vi "Dark Sky Time Machine Request.vi"(0 "API Key":string, 1 "Units":T4="auto", 5 "Latitude":dbl=42.3601 min=-90.0 max=90.0, 7 "Longitude":dbl=-71.0589 min=-180.0 max=180.0, 9 "Time Machine Date/Time":timestamp=timestamp(3584408400 s since 1904-01-01), 11 "error in":errorcluster, 12 "Language":T5=enum."English") -> (4 "Time Machine Forecast Output":T3 {"Current Data"."currently"."time" format="%#_10g"}, 15 "error out":errorcluster)   [LabVIEW 2017, in "Dark Sky Weather Data for LabVIEW.lvlib"]
doc: "Makes a Time Machine request to the DarkSky API and interprets the result. A Time Machine request returns the observed (in the past) or forecasted (in the future) hour-by-hour weather and daily weather conditions for a particular date. Results include the overall data for the day, data by the hour of that day, and the current data for the specific minute, of the request, in that day.\n\nThis API call requires an API key (available free from DarkSky), latitude + longitude coordinates, and a date/time which can be in the past, present, or future. Use this alongside another API, for example from Google, to convert city names into coordinates if needed.\n\nMore info at https://darksky.net/dev/docs/time-machine\n\nNeed an API Key? Visit: https://darksky.net/dev/ and sign up for free!"
uses:
  Dark Sky Weather Data for LabVIEW.lvlib
  Controls/Language Enum.ctl
  Controls/Units Enum.ctl
  Controls/Lat_Lon_TZ.ctl
  Controls/Forecast Current Data.ctl
  <vilib>/httpClient/LabVIEWHTTPClient.lvlib
panel:
  out "API Call URL":string
  # "Inputs"
  # "Outputs - More Info at https://darksky.net/dev/docs/time-machine"
  # "Powered by Dark Sky"
  # "Need an API Key? Visit:\nhttps://darksky.net/dev/\nand sign up for free!"
  # "Instructions:\n-Enter an API Key\n-Enter Longitude, Latitude\n-Enter a Past UNIX Time\n-Run the VI"
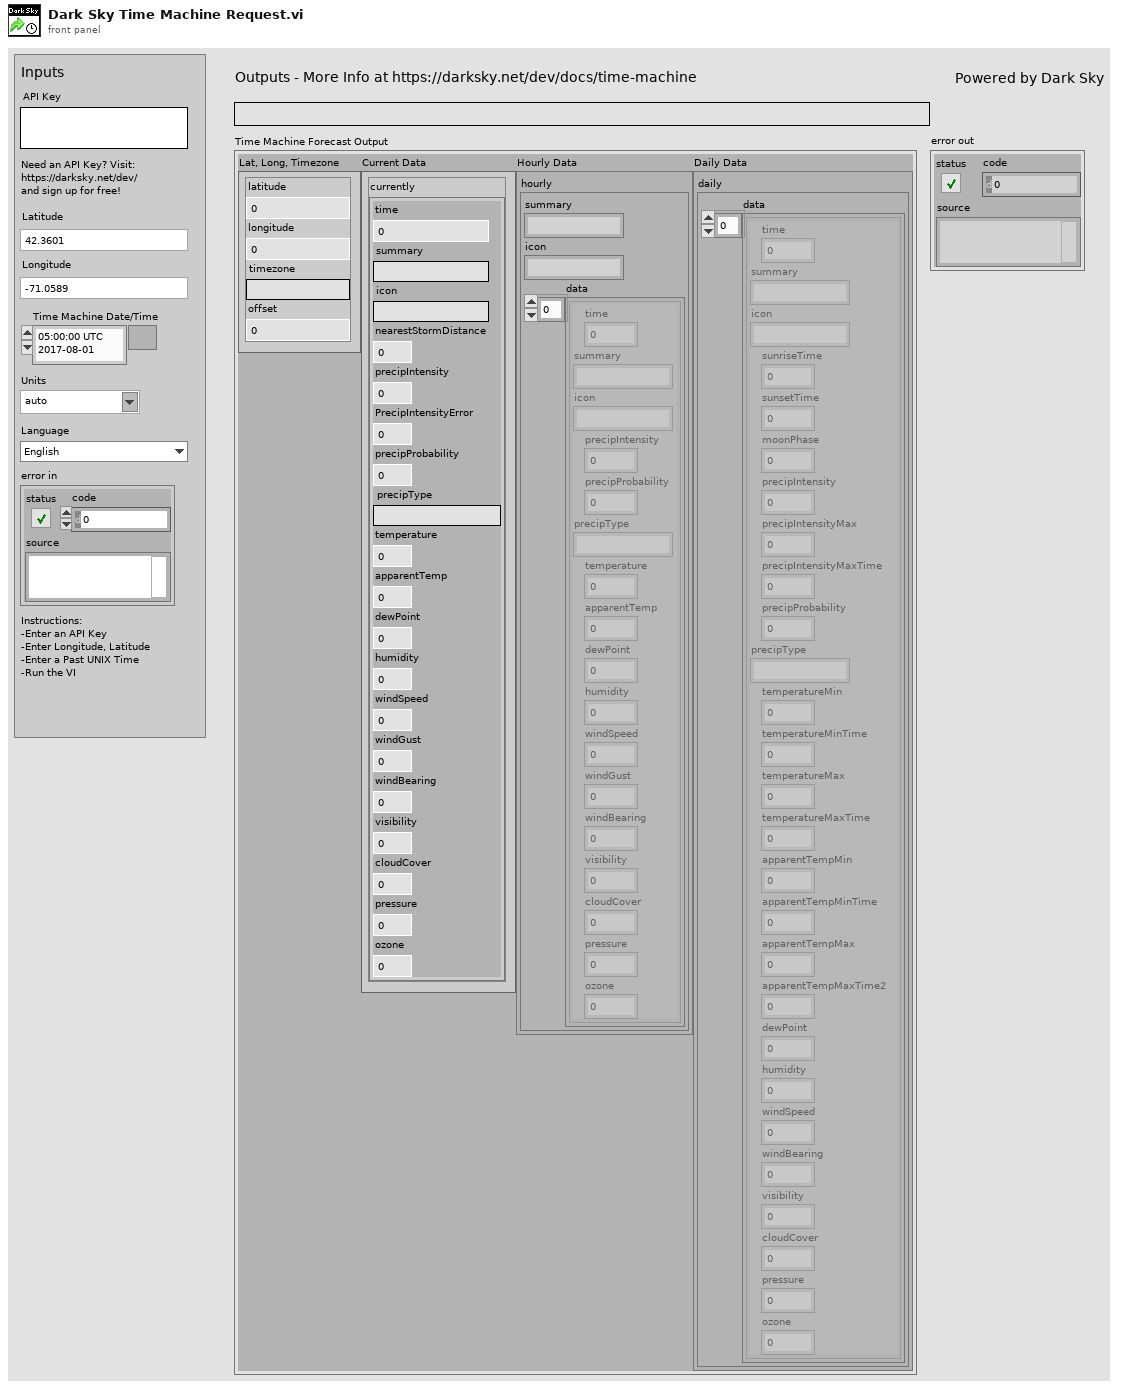
[diagram p1: front panel]
types:
  T1 = typedef "Dark Sky Weather Data for LabVIEW.lvlib/Lat_Lon_TZ.ctl" = cluster{"latitude":dbl, "longitude":dbl, "timezone":string, "offset":dbl}
  T2 = typedef "Dark Sky Weather Data for LabVIEW.lvlib/Forecast Current Data.ctl" = cluster{"currently":cluster{"time":dbl, "summary":string, "icon":string, "nearestStormDistance":dbl, "precipIntensity":dbl, "PrecipIntensityError":dbl, "precipProbability":dbl, "precipType":string, "temperature":dbl, "apparentTemp":dbl, "dewPoint":dbl, "humidity":dbl, "windSpeed":dbl, "windGust":dbl, "windBearing":dbl, "visibility":dbl, "cloudCover":dbl, "pressure":dbl, "ozone":dbl}}
  T3 = cluster{"Lat, Long, Timezone":T1, "Current Data":T2, "Hourly Data":cluster{"hourly":cluster{"summary":string, "icon":string, "data":cluster{"time":dbl, "summary":string, "icon":string, "precipIntensity":dbl, "precipProbability":dbl, "precipType":string, "temperature":dbl, "apparentTemp":dbl, "dewPoint":dbl, "humidity":dbl, "windSpeed":dbl, "windGust":dbl, "windBearing":dbl, "visibility":dbl, "cloudCover":dbl, "pressure":dbl, "ozone":dbl}[]}}, "Daily Data":cluster{"daily":cluster{"data":cluster{"time":dbl, "summary":string, "icon":string, "sunriseTime":dbl, "sunsetTime":dbl, "moonPhase":dbl, "precipIntensity":dbl, "precipIntensityMax":dbl, "precipIntensityMaxTime":dbl, "precipProbability":dbl, "precipType":string, "temperatureMin":dbl, "temperatureMinTime":dbl, "temperatureMax":dbl, "temperatureMaxTime":dbl, "apparentTempMin":dbl, "apparentTempMinTime":dbl, "apparentTempMax":dbl, "apparentTempMaxTime2":dbl, "dewPoint":dbl, "humidity":dbl, "windSpeed":dbl, "windBearing":dbl, "visibility":dbl, "cloudCover":dbl, "pressure":dbl, "ozone":dbl}[]}}}
  T4 = typedef "Dark Sky Weather Data for LabVIEW.lvlib/Units Enum.ctl" = string
  T5 = typedef "Dark Sky Weather Data for LabVIEW.lvlib/Language Enum.ctl" = enum16{"Arabic", "Azerbaijani", "Belaursian", "Bulgarian", "Bosnian", "Catalan", "Czech", "German", "Greek", "English", "Spanish", "Estonian", "French", "Croatian", "Hungarian", "Indonesian", "Italian", "Icelandic", "Georgian", "Cornish", "Norwegian Bokmal", "Dutch", "Polish", "Portuguese", "Russian", "Slovak", "Slovenian", "Serbian", "Swedish", "Tetum", "Turkish", "Ukrainian", "simplified Chinese", "traditional Chinese"}
  T6 = typedef "LabVIEWHTTPClient.lvlib/ClientHandle.ctl" = refnum<k1>
  T7 = cluster{"hourly":cluster{"summary":string, "icon":string, "data":cluster{"time":dbl, "summary":string, "icon":string, "precipIntensity":dbl, "precipProbability":dbl, "precipType":string, "temperature":dbl, "apparentTemp":dbl, "dewPoint":dbl, "humidity":dbl, "windSpeed":dbl, "windGust":dbl, "windBearing":dbl, "visibility":dbl, "cloudCover":dbl, "pressure":dbl, "ozone":dbl}[]}}
  T8 = cluster{"daily":cluster{"data":cluster{"time":dbl, "summary":string, "icon":string, "sunriseTime":dbl, "sunsetTime":dbl, "moonPhase":dbl, "precipIntensity":dbl, "precipIntensityMax":dbl, "precipIntensityMaxTime":dbl, "precipProbability":dbl, "precipType":string, "temperatureMin":dbl, "temperatureMinTime":dbl, "temperatureMax":dbl, "temperatureMaxTime":dbl, "apparentTempMin":dbl, "apparentTempMinTime":dbl, "apparentTempMax":dbl, "apparentTempMaxTime2":dbl, "dewPoint":dbl, "humidity":dbl, "windSpeed":dbl, "windBearing":dbl, "visibility":dbl, "cloudCover":dbl, "pressure":dbl, "ozone":dbl}[]}}
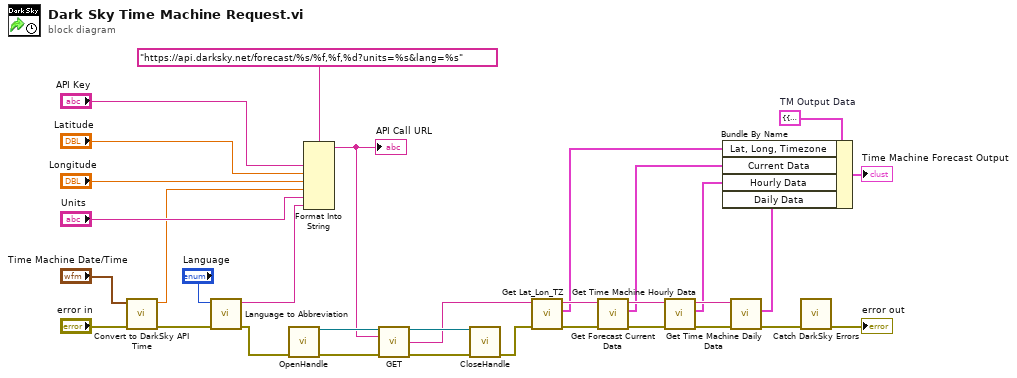
[diagram p0: block diagram]
diagram:
  w12 = T3 {"Lat, Long, Timezone"={"latitude"=0.0, "longitude"=0.0, "timezone"="", "offset"=0.0}, "Current Data"={"currently"={"time"=0.0, "summary"="", "icon"="", "nearestStormDistance"=0.0, "precipIntensity"=0.0, "PrecipIntensityError"=0.0, "precipProbability"=0.0, "precipType"="", "temperature"=0.0, "apparentTemp"=0.0, "dewPoint"=0.0, "humidity"=0.0, "windSpeed"=0.0, "windGust"=0.0, "windBearing"=0.0, "visibility"=0.0, "cloudCover"=0.0, "pressure"=0.0, "ozone"=0.0}}, "Hourly Data"={"hourly"={"summary"="", "icon"="", "data"=[]}}, "Daily Data"={"daily"={"data"=[]}}}  # TM Output Data
  n1 = call "Convert to DarkSky API Time.vi"("error in (no error)"="error in", "Data/Time In"="Time Machine Date/Time") -> ("error out"=w3:errorcluster, "DarkSky Time Out"=w6:dbl)  [unwired: 8 in]
  n2 = call "Language to Abbreviation.vi"("error in (no error)"=w3, "Language"="Language") -> ("error out"=w32:errorcluster, "Language Abbreviation"=w18:string)  [unwired: 8 in]
  n3 = call <vilib>:"OpenHandle.vi"("error in (no error)"=w32) -> ("client handle out"=w25:T6, "error out"=w27:errorcluster)  [unwired: 13 in]
  n4 = Format Into String(format string="https://api.darksky.net/forecast/%s/%f,%f,%d?units=%s&lang=%s", "API Key", "Latitude", "Longitude", w6, "Units", w18) -> (resulting string=w23:string)  [unwired: 2 in, 1 out]
  "API Call URL" <- w23
  n5 = call <vilib>:"GET.vi"("client handle"=w25, "url"=w23, "error in (no error)"=w27) -> ("client handle out"=w24:T6, "body"=w22:string, "error out"=w26:errorcluster)  [unwired: 9 in, 1 out]
  n6 = call <vilib>:"CloseHandle.vi"("client handle"=w24, "error in (no error)"=w26) -> ("error out"=w21:errorcluster)  [unwired: 13 in]
  n7 = call "Get Lat_Lon_TZ.vi"("error in (no error)"=w21, "API Output"=w22) -> ("error out"=w20:errorcluster, "Lat, Long, Timezone"=w8:T1, "API Output (copy)"=w19:string)  [unwired: 7 in]
  n8 = call "Get Forecast Current Data.vi"("error in (no error)"=w20, "API Output"=w19) -> ("error out"=w16:errorcluster, "Current Data"=w9:T2, "API Output (copy)"=w14:string)  [unwired: 7 in]
  n9 = call "Get Time Machine Hourly Data.vi"("error in (no error)"=w16, "API Output"=w14) -> ("error out"=w15:errorcluster, "TM Hourly Data"=w10:T7, "API Output (copy)"=w13:string)  [unwired: 7 in]
  n10 = call "Get Time Machine Daily Data.vi"("error in (no error)"=w15, "API Output"=w13) -> ("error out"=w2:errorcluster, "TM Daily Data"=w11:T8)  [unwired: 7 in, 1 out]
  n11 = Bundle By Name(cluster=w12, "Lat, Long, Timezone"=w8, "Current Data"=w9, "Hourly Data"=w10, "Daily Data"=w11) -> (→"Time Machine Forecast Output":T3)
  n12 = call "Catch DarkSky Errors.vi"("error in (no error)"=w2) -> ("error out"=→"error out":errorcluster)  [unwired: 10 in]
